vi "Hamamatsu_serial.vi"(8 "error in":errorcluster, 9 "IMAQ Session In":refnum<k11>, 10 "Expected Response":string, 11 "Command to send":string) -> (0 "error out":errorcluster, 1 "IMAQ Session Out":refnum<k11>, 3 "Response from Camera":string)   [LabVIEW 2013]
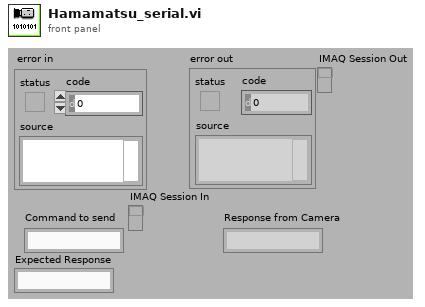
[diagram p1: front panel]
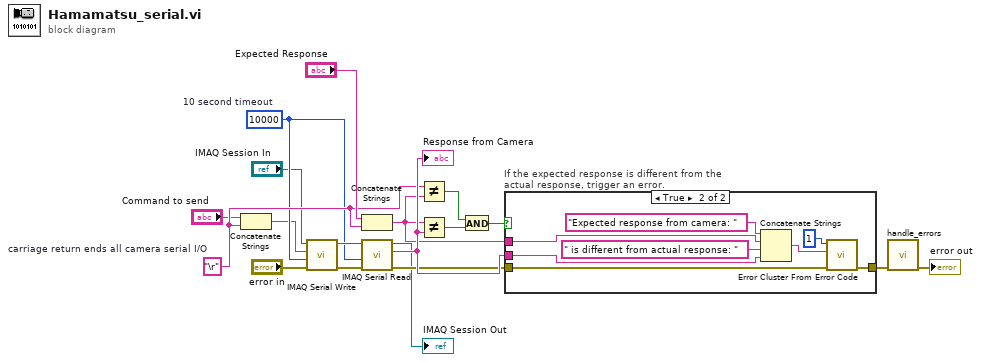
[diagram p0: block diagram]
diagram:
  w12 = "\r"  # carriage return ends all camera serial I/O
  w8 = u32 10000  # 10 second timeout
  n1 = Concatenate Strings("Command to send", w12) -> (w7:string)
  n2 = call <vilib>:"IMAQ Serial Write.vi"("error in (no error)"="error in", "Timeout"=w8, "String to write"=w7, "IMAQ Session In"="IMAQ Session In") -> ("error out"=w11:errorcluster, "IMAQ Session Out"=w10:refnum<k11>)  [unwired: 4 in]
  n3 = Concatenate Strings("Expected Response", w12) -> (w13:string)
  n4 = call <vilib>:"IMAQ Serial Read.vi"("error in (no error)"=w11, "Timeout"=w8, "IMAQ Session In"=w10) -> ("error out"=w9:errorcluster, "String Read"=w15:string, "IMAQ Session Out"=→"IMAQ Session Out":refnum<k11>)  [unwired: 3 in, 1 out]
  "Response from Camera" <- w15
  n5 = Not Equal?(x=w12, y=w13) -> (x != y?=w17:bool)
  n6 = Not Equal?(x=w13, y=w15) -> (x != y?=w18:bool)
  n7 = And(x=w17, y=w18) -> (x .and. y?=w16:bool)
  n8 = case "If the expected response is different from the actual response, trigger an error." shown="True" w16 {
    tunnel: w9 -> [w19 w27]
    tunnel: [w19 w26] -> w2
    tunnel: w13 -> [_ w24]
    tunnel: w15 -> [_ w22]
    frame False {
    }
    frame True {
      n9 = Concatenate Strings("Expected response from camera: " ("string"), w24, " is different from actual response: " ("string"), w22) -> (w21:string)
      n10 = call <vilib>:"Error Cluster From Error Code.vi"("error in (no error)"=w27, "error message (\"\")"=w21, "error code (0)"=1) -> ("error out"=w26:errorcluster)  [unwired: 6 in]
    }
  }
  n11 = call "handle_errors.vi"("error in (no error)"=w2) -> ("error out"=→"error out":errorcluster)  [unwired: 10 in]
